vi "Add First Point.vi"(9 "Accel (f/s^2)":dbl=0.1, 10 "Time (s)":dbl=0.1, 11 "Initial Points":cluster{"x":dbl, "y":dbl, "th":dbl}[](array[cluster])) -> (3 "Points":cluster{"x":dbl, "y":dbl, "th":dbl}[](array[cluster]))   [LabVIEW 2019]
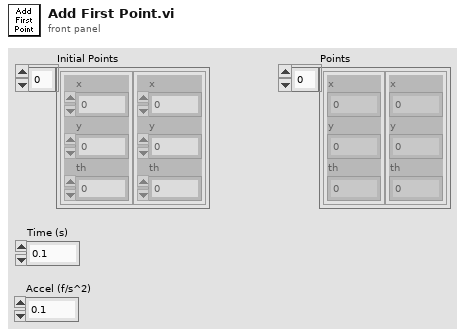
[diagram p1: front panel]
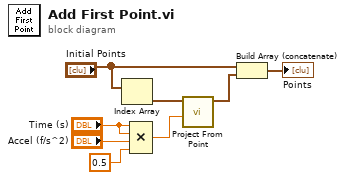
[diagram p0: block diagram]
diagram:
  n1 = Index Array(array="Initial Points") -> (element=w3:cluster{"x":dbl, "y":dbl, "th":dbl})  [unwired: 1 in]
  n2 = Compound Arithmetic op=MULTIPLY("Time (s)", "Time (s)", "Accel (f/s^2)", 0.5) -> (w2:dbl)
  n3 = call "Project From Point.vi"("distance"=w2, "Point In"=w3) -> ("Point Out"=w1:cluster{"x":dbl, "y":dbl, "th":dbl})  [unwired: 9 in]
  n4 = Build Array (concatenate)("Initial Points", w1) -> (→"Points":cluster{"x":dbl, "y":dbl, "th":dbl}[])
